vi "rad_Update Display.vi"(7 "Deployment Notifiers":T1[](array[typedef]), 10 "Stop Updates":refnum<vi>, 11 "Listbox Reference":refnum<vi>) -> ()   [LabVIEW 2023]
uses:
  TypeDefs/rad_Deployment Notifiers.ctl
  TypeDefs/rad_Deployment Status Data Type.ctl
  TypeDefs/rad_Deployment Progress Data Type.ctl
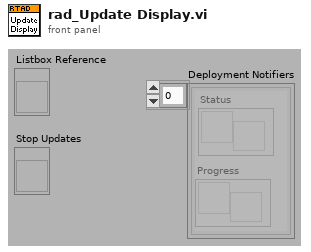
[diagram p1: front panel]
types:
  T1 = typedef "rad_Deployment Notifiers.ctl" = cluster{"Status":refnum<notifier>, "Progress":refnum<notifier>}
  T2 = typedef "rad_Deployment Progress Data Type.ctl" = i8
  T3 = typedef "rad_Deployment Status Data Type.ctl" = string
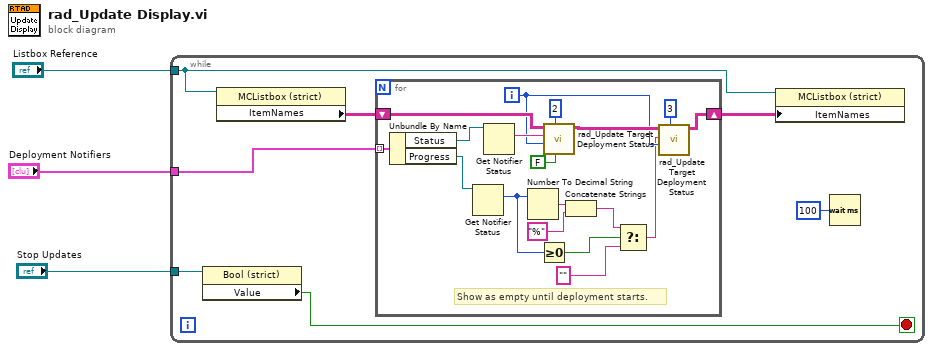
[diagram p0: block diagram]
diagram:
  n1 = while {
    tunnel: "Deployment Notifiers" -> [w10]
    tunnel: "Listbox Reference" -> [w7]
    tunnel: "Stop Updates" -> [w5]
    stop <- w4 stop-if-true
    n2 = property class="Bool (strict)"(reference=w5) -> ("Value"=w4:bool)  [unwired: 1 in, 2 out]
    n3 = property on="Property Node" class="MCListbox (strict)"(reference=w7) -> ("ItemNames"=w8:string[][])  [unwired: 1 in, 2 out]
    n4 = for {
      tunnel: w10 -> [w25] mode=indexing
      shift-right: [w20] -> w9
      shift-left: w8 -> [w27]
      i -> [w16]
      # "Show as empty until deployment starts."
      n5 = Unbundle By Name(w25) -> ("Status"=w24:refnum<notifier>, "Progress"=w22:refnum<notifier>)
      n6 = Get Notifier Status(notifier=w22) -> (current notification=w12:T2)  [unwired: 1 in, 4 out]
      n7 = Get Notifier Status(notifier=w24) -> (current notification=w28:T3)  [unwired: 1 in, 4 out]
      n8 = Number To Decimal String(number=w12) -> (decimal integer string=w18:string)  [unwired: 1 in]
      n9 = Greater Or Equal To 0?(x=w12) -> (x >= 0?=w15:bool)
      n10 = call "rad_Update Target Deployment Status.vi"("Add Timestamp?"=FALSE, "Column"=2, "Target Index"=w16, "Message"=w28, "Targets Deployment Status"=w27) -> ("Targets Deployment Status"=w21:string[][])  [unwired: 6 in]
      n11 = Concatenate Strings(w18, "%" ("string")) -> (w11:string)
      n12 = Select(t=w11, s=w15, f="") -> (s? t:f=w14:string)
      n13 = call "rad_Update Target Deployment Status.vi"("Column"=3, "Target Index"=w16, "Message"=w14, "Targets Deployment Status"=w21) -> ("Targets Deployment Status"=w20:string[][])  [unwired: 7 in]
    }
    n14 = property on="Property Node" class="MCListbox (strict)"(reference=w7, "ItemNames"=w9) -> ()  [unwired: 1 in, 2 out]
    n15 = Wait (ms)(milliseconds to wait=u32 100) -> ()  [unwired: 1 out]
  }
